vi "PH_BlackBox.PC _Calc Position.vi"(0 "i ref in":refnum<vi>, 2 "serviceName":string, 3 "Value":T1 items=["no info", "off/false/out", "on/true/in", "Failure", "Alarm", "Status 1", "Status 2", "Status 3"], 4 "No link":bool, 5 "error in (no error)":errorcluster, 7 "Tip Strip":string="N/A") -> (14 "i ref out":refnum<vi>, 16 "Status changed?":bool, 19 "error out":errorcluster)   [LabVIEW 2014, in "PH_BlackBox.lvlib"]
doc: "This is the action done in the event case \"_CalcPosition\": in case of a change the incoming information is written to own attributes."
uses:
  PH_BlackBox.lvlib
  PH_StatusHandler/PH_StatusHandler.Status.ctl
  PH_Common/PH_Common.lvlib
  PH_Beckhoff_Common/PH_Beckhoff_Common.lvlib
  PH_StatusHandler/PH_StatusHandler.lvlib
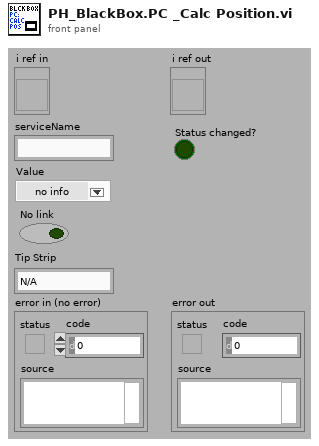
[diagram p1: front panel]
types:
  T1 = typedef "PH_StatusHandler.lvlib/PH_StatusHandler.Status.ctl" = i16
  T2 = typedef "PH_BlackBox.lvlib/PH_BlackBox.i attribute.ctl" = cluster{"BB Remote Controlled?":bool, "GUI Refs":T3, "Position IN":T1, "Position OUT":T1, "BB Remote Controlled by other Instance?":bool, "Recipient":string, "Number":i32, "Caption Move":string, "Caption Out":string, "Caption In":string}
  T3 = typedef "PH_BlackBox.lvlib/PH_BlackBox.GUI Refs.ctl" = cluster{"MOVE IN":refnum<vi>, "MOVE":refnum<vi>, "IN":refnum<vi>, "OUT":refnum<vi>, "REMOTE":refnum<vi>, "GUI-Knob Move":refnum<vi>, "GUI-Knob Move in":refnum<vi>, "POWER ON":refnum<vi>, "Delete":refnum<vi>, "Function Textfield":refnum<vi>}
  T4 = typedef "PH_Beckhoff_Common.lvlib/PH_Beckhoff_Common.BB Tagnames.ctl" = cluster{"Sensor Remote controlled":string, "Sensor Out":string, "Sensor In":string, "Actor Direction In":string, "Actor Move":string, "Sensor Power ok":string, "Instance":string}
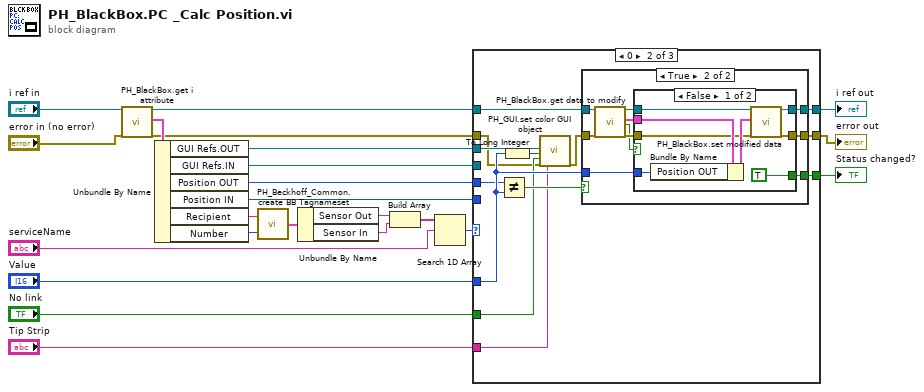
[diagram p0: block diagram]
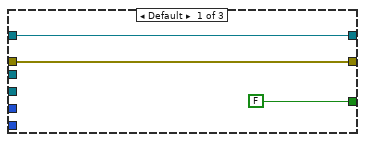
[diagram p2: hidden frame]
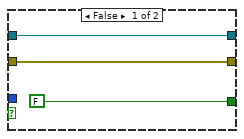
[diagram p3: hidden frame]
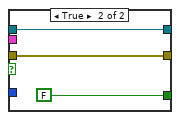
[diagram p4: hidden frame]
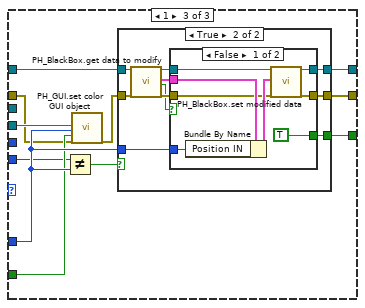
[diagram p5: hidden frame]
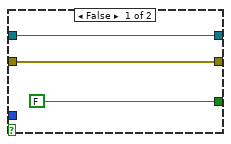
[diagram p6: hidden frame]
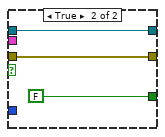
[diagram p7: hidden frame]
diagram:
  n1 = call "PH_BlackBox.get i attribute.vi"("i ref in"="i ref in", "error in (no error)"="error in (no error)") -> ("i ref out"=w9:refnum<vi>, "i attribute"=w13:T2, "error out"=w8:errorcluster)  [unwired: 15 in]
  n2 = Unbundle By Name(w13) -> ("GUI Refs.OUT"=w7:refnum<vi>, "GUI Refs.IN"=w5:refnum<vi>, "Position OUT"=w6:T1, "Position IN"=w4:T1, "Recipient"=w3:string, "Number"=w2:i32)
  n3 = call "PH_Beckhoff_Common.create BB Tagnameset.vi"("#"=w2, "Instance Name"=w3) -> ("output cluster"=w12:T4)
  n4 = Unbundle By Name(w12) -> ("Sensor Out"=w11:string, "Sensor In"=w10:string)
  n5 = Build Array(w11, w10) -> (w20:string[])
  n6 = Search 1D Array(1D array=w20, element="serviceName") -> (index of element=w18:i32)  [unwired: 1 in]
  n7 = case shown="0" w18 {
    tunnel: [w25 w38 w73] -> w23
    tunnel: [w26 w39 w74] -> w22
    tunnel: "Value" -> [_ w34 w69]
    tunnel: w8 -> [w25 w29 w64]
    tunnel: w9 -> [w26 w30 w65]
    tunnel: [FALSE w36 w71] -> w17
    tunnel: "No link" -> [_ w33 w68]
    tunnel: w7 -> [_ w32 _]
    tunnel: w6 -> [_ w31 _]
    tunnel: w5 -> [_ _ w67]
    tunnel: w4 -> [_ _ w66]
    tunnel: "Tip Strip" -> [_ w27 _]
    frame Default {
    }
    frame 0 {
      n8 = Not Equal?(x=w31, y=w34) -> (x != y?=w37:bool)
      n9 = To Long Integer(number=w34) -> (32bit integer=w28:i32)
      n10 = call "PH_GUI.set color GUI object.vi"("GUI object Ref"=w32, "State"=w28, "Blinking? (false)"=w33, "error in (no error)"=w29, "Tip Strip (N/A)"=w27) -> ("error out"=w35:errorcluster)  [unwired: 14 in]
      n11 = case shown="True" w37 {
        tunnel: [w42 w48] -> w39
        tunnel: [w41 w47] -> w38
        tunnel: w35 -> [w41 w46]
        tunnel: w30 -> [w42 w45]
        tunnel: w34 -> [_ w44]
        tunnel: [FALSE w43] -> w36
        frame False {
        }
        frame True {
          n12 = call "PH_BlackBox.get data to modify.vi"("i ref in"=w45, "error in (no error)"=w46) -> ("i ref out"=w51:refnum<vi>, "i attribute"=w49:T2, "timed out"=w50:bool, "error out"=w52:errorcluster)  [unwired: 14 in]
          n13 = case shown="False" w50 {
            tunnel: w52 -> [w53 w62]
            tunnel: [w60 w62] -> w47
            tunnel: w51 -> [w59 w63]
            tunnel: [w58 w63] -> w48
            tunnel: w49 -> [w57 _]
            tunnel: w44 -> [w55 _]
            tunnel: [TRUE FALSE] -> w43
            frame False {
              n14 = Bundle By Name(cluster=w57, "Position OUT"=w55) -> (w56:T2)
              n15 = call "PH_BlackBox.set modified data.vi"("i ref in"=w59, "i attribute"=w56, "error in (no error)"=w53) -> ("i ref out"=w58:refnum<vi>, "error out"=w60:errorcluster)  [unwired: 15 in]
            }
            frame True {
            }
          }
        }
      }
    }
    frame 1 {
      n16 = Not Equal?(x=w66, y=w69) -> (x != y?=w72:bool)
      n17 = call "PH_GUI.set color GUI object.vi"("GUI object Ref"=w67, "State"=w69, "Blinking? (false)"=w68, "error in (no error)"=w64) -> ("error out"=w70:errorcluster)  [unwired: 15 in]
      n18 = case shown="True" w72 {
        tunnel: [w77 w83] -> w74
        tunnel: [w76 w82] -> w73
        tunnel: w70 -> [w76 w81]
        tunnel: w65 -> [w77 w80]
        tunnel: w69 -> [_ w79]
        tunnel: [FALSE w78] -> w71
        frame False {
        }
        frame True {
          n19 = call "PH_BlackBox.get data to modify.vi"("i ref in"=w80, "error in (no error)"=w81) -> ("i ref out"=w86:refnum<vi>, "i attribute"=w84:T2, "timed out"=w85:bool, "error out"=w87:errorcluster)  [unwired: 14 in]
          n20 = case shown="False" w85 {
            tunnel: w87 -> [w88 w97]
            tunnel: [w95 w97] -> w82
            tunnel: w86 -> [w94 w98]
            tunnel: [w93 w98] -> w83
            tunnel: w84 -> [w92 _]
            tunnel: w79 -> [w90 _]
            tunnel: [TRUE FALSE] -> w78
            frame False {
              n21 = Bundle By Name(cluster=w92, "Position IN"=w90) -> (w91:T2)
              n22 = call "PH_BlackBox.set modified data.vi"("i ref in"=w94, "i attribute"=w91, "error in (no error)"=w88) -> ("i ref out"=w93:refnum<vi>, "error out"=w95:errorcluster)  [unwired: 15 in]
            }
            frame True {
            }
          }
        }
      }
    }
  }
  "error out" <- w23
  "i ref out" <- w22
  "Status changed?" <- w17
